vi "Create Text.vi"(8 "error in (no error)":errorcluster, 9 "Color":T1={"Red"=1.0, "Green"=0.0, "Blue"=0.0, "Alpha"=1.0}, 10 "Path to font file":path, 11 "Text":string) -> (0 "error out":errorcluster, 3 "New Text Refnum":refnum<vi>)   [LabVIEW 2017, in "NI_3D Picture Control.lvlib"]
doc: "Sets a 3D object you create with the Create Object VI to a text object and applies the text, font, and color you specify to the object."
uses:
  <vilib>/picture/3D Picture Control/NI_3D Picture Control.lvlib
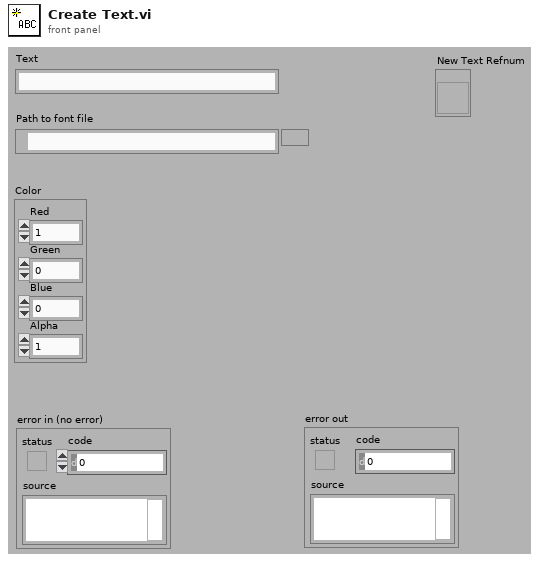
[diagram p1: front panel]
types:
  T1 = cluster{"Red":sgl, "Green":sgl, "Blue":sgl, "Alpha":sgl}
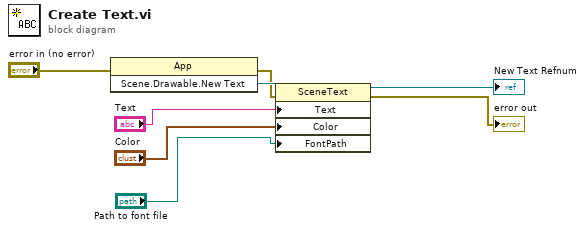
[diagram p0: block diagram]
diagram:
  n1 = invoke class="App" method="Scene.Drawable.New Text"(error in="error in (no error)") -> (error out=w1:errorcluster, "Scene.Drawable.New Text"=w8:refnum<vi>)  [unwired: 2 in, 1 out]
  n2 = property class="SceneText"(reference=w8, error in=w1, "Text"="Text", "Color"="Color", "FontPath"="Path to font file") -> (reference out=→"New Text Refnum":refnum<vi>, error out=→"error out":errorcluster)
